vi "RngFind_Logger.vi"(0 "4145_GPIB_COM_ctrl":T2={"Address_string"="17", "timeout ms"=25000, "Terminator"=",", "LoggerQueue"=refnum}, 1 "msg":string, 2 "msg_type":T1, 3 "origin vi":string, 7 "error in (no error)":errorcluster) -> (8 "error out":errorcluster)   [LabVIEW 2014]
uses:
  4145_Data_Util_code_ver_1.1/4145_Data_Util/typedef/4145_GPIB_Com.ctl
  4145_Data_Util_code_ver_1.1/4145_Data_Util/typedef/4145_que_msg.ctl
  4145_Data_Util_code_ver_1.1/4145_Data_Util/typedef/4145 command enum.ctl
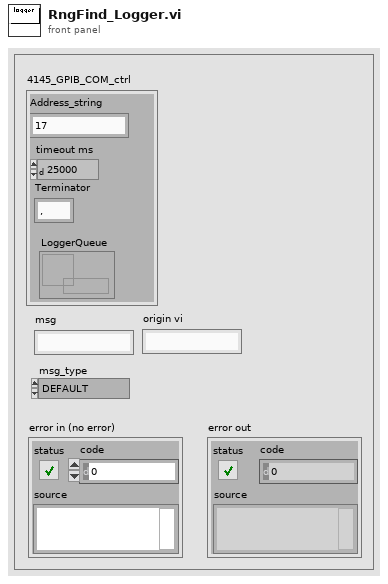
[diagram p1: front panel]
types:
  T1 = typedef "4145 command enum.ctl" = enum16{"DEFAULT", "INFORMATION", "ERROR", "STATUS", "CAUTION", "WARNING", "OFFLINE", "STOP"}
  T2 = typedef "4145_GPIB_Com.ctl" = cluster{"Address_string":string, "timeout ms":u32, "Terminator":string, "LoggerQueue":refnum<queue>}
  T3 = typedef "4145_que_msg.ctl" = cluster{"msg":string, "msg_type":T1}
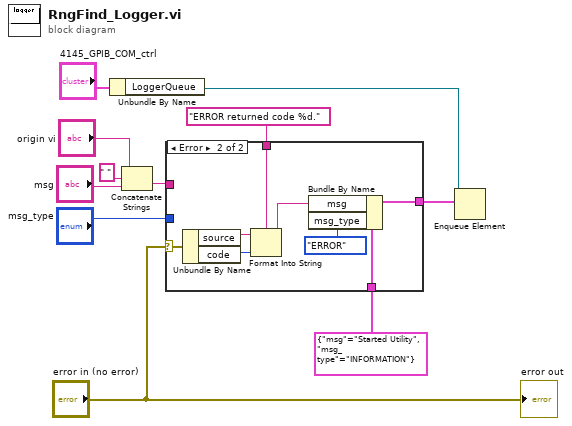
[diagram p0: block diagram]
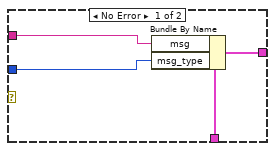
[diagram p2: hidden frame]
diagram:
  n1 = Unbundle By Name("4145_GPIB_COM_ctrl") -> ("LoggerQueue"=w10:refnum<queue>)
  n2 = Concatenate Strings("origin vi", " " ("string"), "msg") -> (w2:string)
  n3 = case shown="Error" "error in (no error)" {
    selector: "error in (no error)" -> [_ w23]
    tunnel: T3 {"msg"="Started Utility", "msg_type"=enum."INFORMATION"} ("4145_que_msg") -> [w15 w22]
    tunnel: [w14 w21] -> w8
    tunnel: "msg_type" -> [w13 _]
    tunnel: w2 -> [w12 _]
    tunnel: "ERROR returned code %d." -> [_ w19]
    frame No Error {
      n4 = Bundle By Name(cluster=w15, "msg"=w12, "msg_type"=w13) -> (w14:T3)
    }
    frame Error {
      n5 = Unbundle By Name(w23) -> ("source"=w17:string, "code"=w18:i32)
      n6 = Format Into String(format string=w19, initial string=w17, w18) -> (resulting string=w16:string)  [unwired: 1 in, 1 out]
      n7 = Bundle By Name(cluster=w22, "msg"=w16, "msg_type"=4145_command_enum."ERROR") -> (w21:T3)
    }
  }
  n8 = Enqueue Element(queue=w10, element=w8) -> ()  [unwired: 2 in, 3 out]
  "error out" <- "error in (no error)"
